vi "FdxCmdTxVLControlCvi.vi"(8 "error in":errorcluster, 9 "TxVLControl":cluster{"VlId":u32, "EnableTyp":u32} {"EnableTyp" items=["FDX_DIS", "FDX_ENA"]}, 11 "InstrumentHandle":u32) -> (0 "error out":errorcluster, 3 "InstrumentHandle":u32)   [LabVIEW 2020, in "AIM664LV.lvlib"]
doc: "This function is used to enable or disable a VL. By default all VL’s are enabled. For Individual\nTransmit Mode each VL must be explicitly created with the function FdxCmdTxCreateVL or\nFdxCmdTxCreateHiResVL."
uses:
  AIM664LV.lvlib
  AFDX_LibraryAdmin/FdxGlobalDllPath.vi
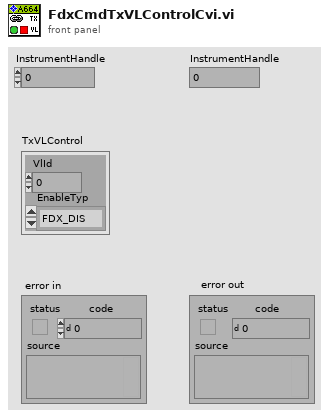
[diagram p1: front panel]
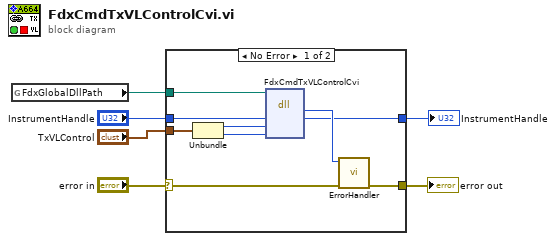
[diagram p0: block diagram]
diagram:
  n1 = global read "FdxGlobalDllPath.vi" "FdxGlobalDllPath"() -> (w4:path)
  n2 = case shown="No Error" "error in" {
    selector: "error in" -> [w14 w17]
    tunnel: [w15 w17] -> w6
    tunnel: w4 -> [w10 _]
    tunnel: "TxVLControl" -> [w9 _]
    tunnel: "InstrumentHandle" -> [w8 w16]
    tunnel: [w7 w16] -> w1
    frame No Error {
      n3 = Unbundle(w9) -> ("VlId"=w12:u32, "EnableTyp"=w11:u32)
      n4 = dll-call lib="aim_fdx.19.dll" fn="FdxCmdTxVLControlCvi"(path in=w10, "InstrumentHandle"=w8, "VlId"=w12, "EnableTyp"=w11) -> ("status"=w13:i32, "InstrumentHandle"=w7:u32)  [unwired: 4 in, 2 out]
      n5 = call "ErrorHandler.vi"("error in"=w14, "AIM Error"=w13) -> ("error out"=w15:errorcluster)  [unwired: 9 in]
    }
    frame Error {
    }
  }
  "error out" <- w6
  "InstrumentHandle" <- w1
